vi "output.vi"(8 "error in":errorcluster, 10 "data table in":T1, 11 "EthernetIP runtime in":refnum<class "EthernetIP runtime.lvclass">) -> (0 "error out":errorcluster, 2 "data table out":T1, 3 "EthernetIP runtime out":refnum<class "EthernetIP runtime.lvclass">)   [LabVIEW 2013, in "EthernetIP runtime.lvclass"]
doc: "Provides an interface for writing data to a module at runtime. While this interface performs no operations, a child should provide an override which may write to any open sessions, references, or interfaces."
uses:
  EthernetIP runtime.lvclass
  <vilib>/NI/Tag Bus/table/data table.ctl
  EthernetIP runtime.lvclass/EthernetIP runtime.ctl
  <vilib>/ethernetip/ethernetip.lvlib
  <vilib>/NI/Tag Bus/table/data table.lvlib
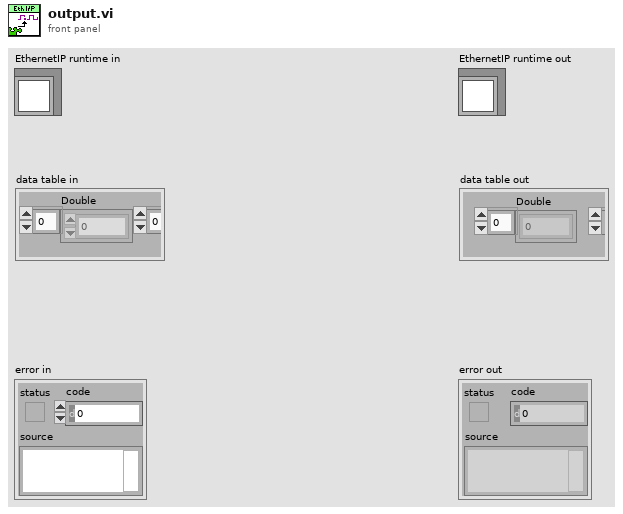
[diagram p1: front panel]
types:
  T1 = typedef "tag bus.lvlib/data table.lvlib/data table.ctl" = cluster{"Double":dbl[], "Single":sgl[], "I64":i64[], "I32":i32[], "I16":i16[], "I8":i8[], "U64":u64[], "U32":u32[], "U16":u16[], "U8":u8[], "Boolean":bool[], "String":string[], "Array of Double":cluster{"DBL Array":dbl[]}[], "Array of Single":cluster{"SGL Array":sgl[]}[], "Array of I64":cluster{"I64 Array":i64[]}[], "Array of I32":cluster{"I32 Array":i32[]}[], "Array of I16":cluster{"I16 Array":i16[]}[], "Array of I8":cluster{"I8 Array":i8[]}[], "Array of U64":cluster{"U64 Array":u64[]}[], "Array of U32":cluster{"U32 Array":u32[]}[], "Array of U16":cluster{"U16 Array":u16[]}[], "Array of U8":cluster{"U8 Array":u8[]}[], "Array of Boolean":cluster{"Boolean Array":bool[]}[], "Array of String":cluster{"String Array":string[]}[]}
  T2 = typedef "ethernetip.lvlib/ethernetip.ctl" = refnum<k21>
  T3 = typedef "EthernetIP runtime.lvclass/assembly data spec.ctl" = cluster{"Instance ID":u32, "specification":T4[], "big endian?":bool}
  T4 = typedef "EthernetIP runtime.lvclass/conversion specification.ctl" = cluster{"data type":T5, "data index":i32, "byte index":i32, "subindex/len":i32}
  T5 = typedef "tag bus.lvlib/tag descriptor.lvclass/Data Type.ctl" = enum16{"Double", "Single", "I64", "I32", "I16", "I8", "U64", "U32", "U16", "U8", "Boolean", "String", "Array of Double", "Array of Single", "Array of I64", "Array of I32", "Array of I16", "Array of I8", "Array of U64", "Array of U32", "Array of U16", "Array of U8", "Array of Boolean", "Array of String"}
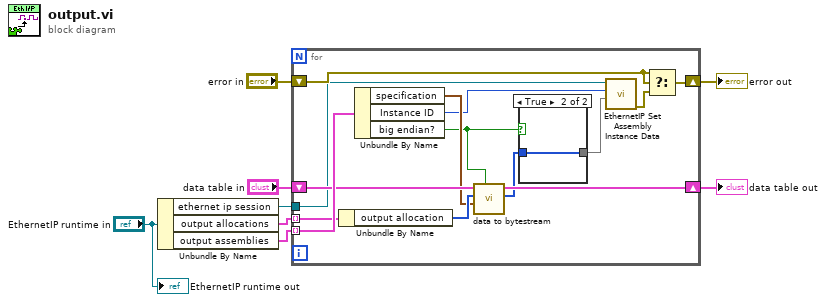
[diagram p0: block diagram]
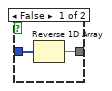
[diagram p2: hidden frame]
diagram:
  n1 = Unbundle By Name("EthernetIP runtime in") -> ("ethernet ip session"=w8:T2, "output allocations"=w1:cluster{"output allocation":u8[]}[], "output assemblies"=w7:T3[])
  n2 = for {
    tunnel: w8 -> [w14]
    shift-right: [w21] -> w5
    shift-left: "error in" -> [w22]
    tunnel: w7 -> [w20] mode=indexing
    shift-right: [w13] -> w3
    shift-left: "data table in" -> [w19]
    tunnel: w1 -> [w18] mode=indexing
    n3 = Unbundle By Name(w18) -> ("output allocation"=w17:u8[])
    n4 = Unbundle By Name(w20) -> ("specification"=w16:T4[], "Instance ID"=w12:u32, "big endian?"=w9:bool)
    n5 = call "data to bytestream.vi"("big endian?"=w9, "specifications"=w16, "byte allocation"=w17, "data table"=w19) -> ("bytestream"=w11:u8[], "allocation"=w13:T1)  [unwired: 6 in]
    n6 = case shown="True" w9 {
      tunnel: [w23 w25] -> w10
      tunnel: w11 -> [w24 w25]
      frame False {
        n7 = Reverse 1D Array(array=w24) -> (reversed array=w23:u8[])
      }
      frame True {
      }
    }
    n8 = call <vilib>:"EthernetIP Set Assembly Instance Data.vi"("Data"=w10, "Instance ID in"=w12, "Session in"=w14) -> ("error out"=w15:errorcluster)  [unwired: 6 in, 2 out]
    n9 = Select(t=w22, s=w22, f=w15) -> (s? t:f=w21:errorcluster)
  }
  "error out" <- w5
  "data table out" <- w3
  "EthernetIP runtime out" <- "EthernetIP runtime in"
